vi "Verify Person as JSON.vi"(8 "error in":errorcluster) -> (0 "error out":errorcluster)   [LabVIEW 2020, in "Caraya Extension Tests.lvclass"]
uses:
  Caraya Extension Tests.lvclass
  Common/Person/Person.lvclass
  Common/Person/Person.lvclass/Person.ctl
  Common/Person/Write First Name.vi
  Common/Person/Write Last Name.vi
  Common/Person/Write Title.vi
  <vilib>/addons/_JKI Toolkits/Caraya/classes/Test/Test.lvclass
  Source/Extensions/Caraya.Extension/Caraya.Extension.lvlib
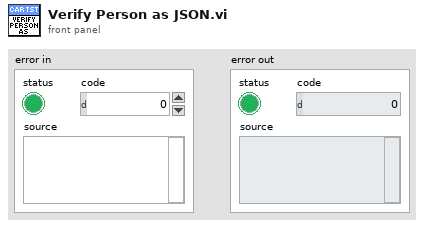
[diagram p1: front panel]
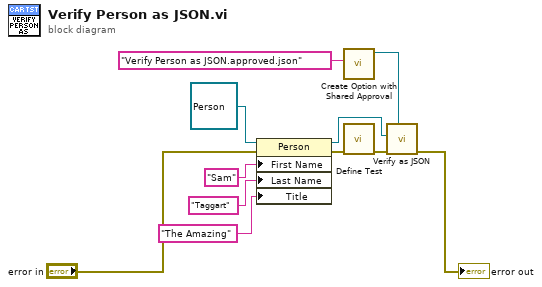
[diagram p0: block diagram]
diagram:
  n1 = property on="Property Node" class="Person"(reference=refnum<class "Person.lvclass"> refnum ("Person.lvclass"), error in="error in", "First Name"="Sam", "Last Name"="Taggart", "Title"="The Amazing") -> (reference out=w3:refnum<class "Person.lvclass">, error out=w8:errorcluster)
  n2 = call "Create Option with Shared Approval.vi"("Filename"="Verify Person as JSON.approved.json") -> ("Options outs"=w1:refnum<class "Options.lvclass">)  [unwired: 10 in]
  n3 = call <vilib>:"Define Test.vi"("error in (no error)"=w8) -> ("error out"=w11:errorcluster)  [unwired: 9 in, 1 out]
  n4 = call "Verify as JSON.vi"("Options"=w1, "error in"=w11, "Anything"=w3) -> ("error out"=→"error out":errorcluster)  [unwired: 7 in, 1 out]
